vi "Receive U32 Value Msg.vi"(8 "error in (no error)":errorcluster, 10 "U32ValueMsg":refnum<class "U32ValueMsg.lvclass">, 11 "IViewable in":refnum<class "IViewable.lvclass">) -> (0 "error out":errorcluster, 3 "IViewable out":refnum<class "IViewable.lvclass">)   [LabVIEW 2015, in "IViewable.lvlib" / "IViewable.lvclass"]
uses:
  IViewable.lvclass
  AutoRegistration/ActorAutoRegistration Messages/U32ValueMsg/U32ValueMsg.lvclass
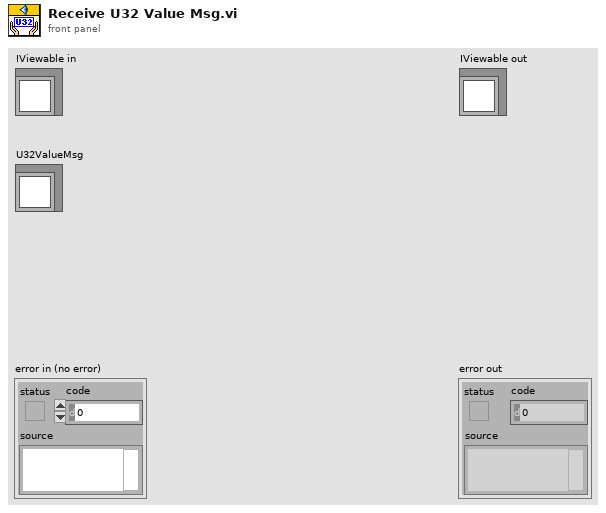
[diagram p1: front panel]
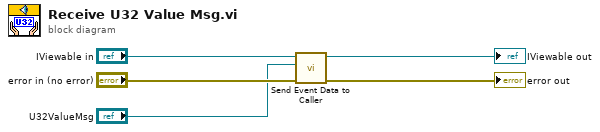
[diagram p0: block diagram]
diagram:
  n1 = call "Send Event Data to Caller.vi"("error in (no error)"="error in (no error)", "EventDataMsg"="U32ValueMsg", "IViewable in"="IViewable in") -> ("error out"=→"error out":errorcluster, "IViewable out"=→"IViewable out":refnum<class "IViewable.lvclass">)  [unwired: 7 in]
